vi "UnitTest.vi"() -> ()   [LabVIEW 2018]
doc: "This VI Tests the movement, and control of the Thorlab Axis Controller. You can use it to send any kind of configuration, or list of commands and verify things work properly.\n\nCreator: Slade Jeppesen\nCreated: 09/30/20"
uses:
  PPLs/Axis/Parent/Axis.lvlibp/Custom Controls/Command.ctl
  Thorlabs.lvclass
  PPLs/Axis/Parent/Axis.lvlibp/Custom Controls/Jog Direction.ctl
  PPLs/Axis/Parent/Axis.lvlibp/Axis.lvclass
  PPLs/Axis/Parent/Axis.lvlibp
  C:/AME Test Engineering/LabVIEW/PPLs/Axis/Parent/Axis.lvlibp/Axis.lvclass
panel:
  in  "PPLs Folder Path":path
  in  "INI File Path":path
  in  "Stop":bool
  in  "Jog Forwad":bool
  in  "Jog Back":bool
  in  "Step Back":bool
  in  "Step Forward":bool
  out "Error Out":errorcluster
  in  "Error In":errorcluster
  out "Current Position":dbl
  in  "Value":dbl
  out "Homed?":bool
  out "Moving?":bool
  out "Home Success?":bool
  in  "Command":T1
  in  "Home":bool
  in  "SendCMD":bool
  in  "Device":string
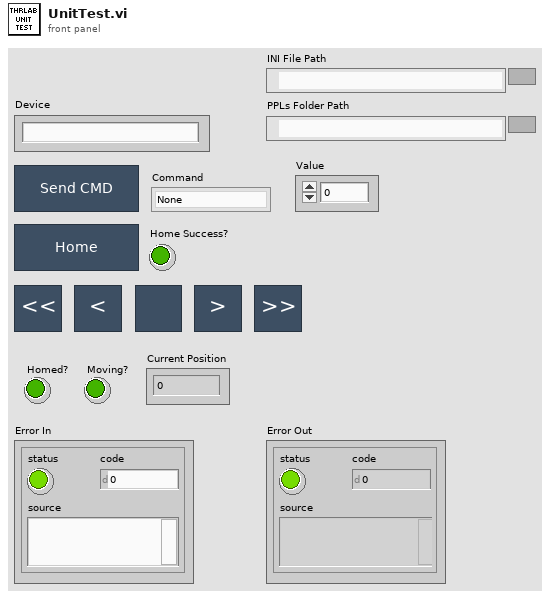
[diagram p1: front panel]
types:
  T1 = typedef "Axis.lvlibp/Command.ctl" = enum16{"None", "Home", "Renumber", "Move Absolute", "Move Relative", "Stop", "Set Run Speed", "Set Acceleration", "Set Run Current", "Set Home Offset", "Set Home Speed", "Query Current Position", "Load Defaults", "Query Status", "Lock Controls", "Unlock Controls", "Set Jog Step Size", "Set Jog Acceleration", "Set Jog Speed", "Query Homed Status", "Query Moving Status", "Reset", "Set Max Position", "Set Min Position"}
  T2 = typedef "Axis.lvlibp/Jog Direction.ctl" = enum16{"Forward", "Backward"}
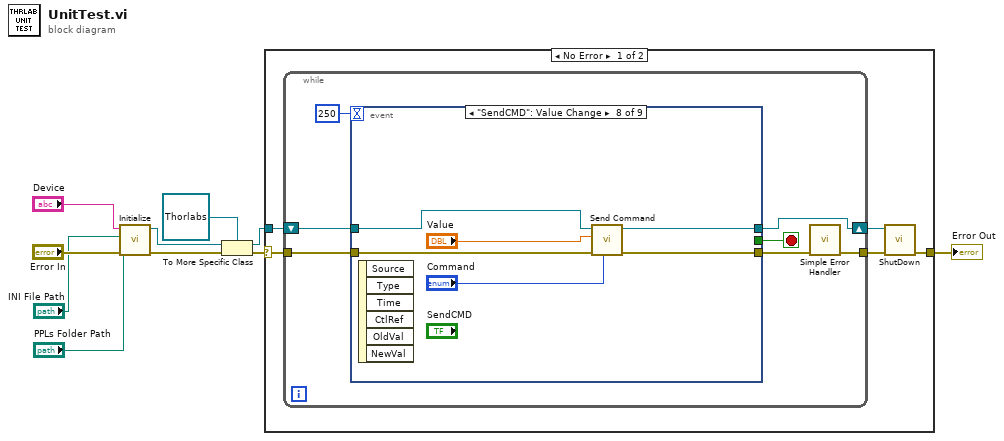
[diagram p0: block diagram]
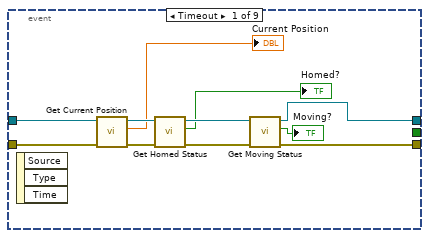
[diagram p2: hidden frame]
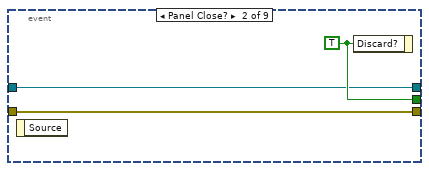
[diagram p3: hidden frame]
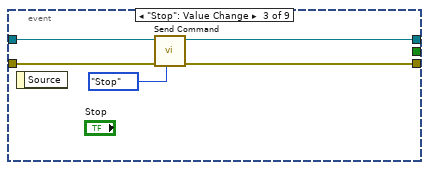
[diagram p4: hidden frame]
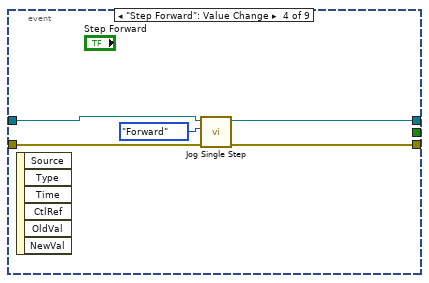
[diagram p5: hidden frame]
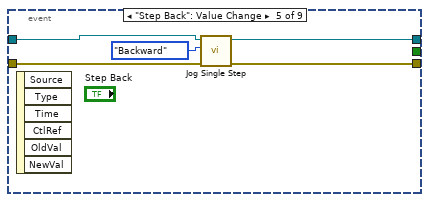
[diagram p6: hidden frame]
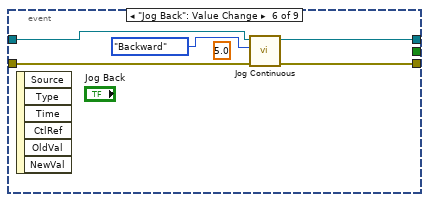
[diagram p7: hidden frame]
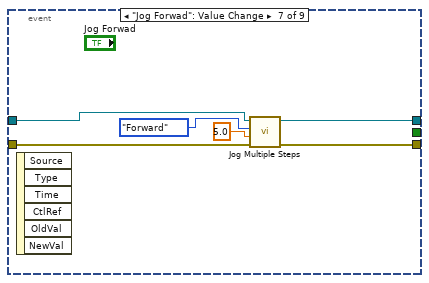
[diagram p8: hidden frame]
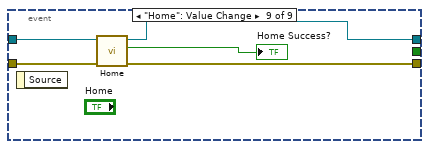
[diagram p9: hidden frame]
diagram:
  n1 = call "Initialize.vi"("error in"="Error In", "PPLs Folder Path"="PPLs Folder Path", "INI File Path"="INI File Path", "Device"="Device") -> ("error out"=w8:errorcluster, "Axis out"=w10:refnum<class "Axis.lvclass">)  [unwired: 6 in]
  n2 = To More Specific Class(target class=refnum<class "Thorlabs.lvclass"> refnum ("Thorlabs.lvlib:Thorlabs.lvclass"), reference=w10, error in=w8) -> (specific class reference=w7:refnum<class "Thorlabs.lvclass">, error out=w6:errorcluster)
  n3 = case shown="No Error" w6 {
    selector: w6 -> [w11 w74]
    tunnel: w7 -> [w15 _]
    tunnel: [w13 w74] -> w4
    frame No Error {
      n4 = while {
        shift-right: [w19] -> w14
        shift-left: w15 -> [w20]
        tunnel: w11 -> [w21]
        tunnel: [w17] -> w12
        stop <- w22 stop-if-true
        n5 = event shown="[7] \"SendCMD\": Value Change" {
          selector: _ -> [_ _ _ _ _ _ _ _ _]
          dyn-events: _ -> [_ _ _ _ _ _ _ _ _]
          timeout: 250 -> [_ _ _ _ _ _ _ _ _]
          tunnel: [_ w36 _ _ _ _ _ _ _] -> w22
          tunnel: w21 -> [w26 w34 w40 w46 w51 w55 w59 w65 w73]
          tunnel: w20 -> [w23 w35 w37 w45 w50 w52 w60 w68 w72]
          tunnel: [w24 w35 w38 w43 w49 w53 w57 w67 w71] -> w19
          tunnel: [w25 w34 w39 w42 w48 w54 w58 w66 w70] -> w18
          event Timeout {
            n6 = event-data() -> ()  [unwired: 1 in, 3 out]
            n7 = call "Get Current Position.vi"("error in"=w26, "Axis in"=w23) -> ("error out"=w31:errorcluster, "Current Position"=→"Current Position":dbl, "Axis out"=w33:refnum<class "Thorlabs.lvclass">)  [unwired: 7 in]
            n8 = call "Get Homed Status.vi"("error in (no error)"=w31, "Axis in"=w33) -> ("error out"=w30:errorcluster, "Homed?"=→"Homed?":bool, "Axis out"=w32:refnum<class "Thorlabs.lvclass">)  [unwired: 7 in]
            n9 = call "Get Moving Status.vi"("error in (no error)"=w30, "Axis in"=w32) -> ("error out"=w25:errorcluster, "Moving?"=→"Moving?":bool, "Axis out"=w24:refnum<class "Thorlabs.lvclass">)  [unwired: 7 in]
          }
          event Panel Close? {
            w36 = TRUE
            n10 = event-data() -> ()  [unwired: 1 in, 1 out]
            n11 = event-data("Discard?"=w36) -> ()  [unwired: 1 in, 1 out]
          }
          event "Stop": Value Change {
            n12 = event-data() -> ()  [unwired: 1 in, 1 out]
            n13 = call-dynamic "Send Command.vi"("Command"=Command."Stop", "error in"=w40, "Thorlabs In"=w37) -> ("error out"=w39:errorcluster, "Thorlabs Out"=w38:refnum<class "Thorlabs.lvclass">)  [unwired: 7 in]
          }
          event "Step Forward": Value Change {
            n14 = event-data() -> ()  [unwired: 1 in, 6 out]
            n15 = call-dynamic "Jog Single Step.vi"("error in (no error)"=w46, "Jog Direction"=Jog_Direction."Forward", "Thorlabs in"=w45) -> ("error out"=w42:errorcluster, "Thorlabs out"=w43:refnum<class "Thorlabs.lvclass">)  [unwired: 7 in]
          }
          event "Step Back": Value Change {
            n16 = event-data() -> ()  [unwired: 1 in, 6 out]
            n17 = call-dynamic "Jog Single Step.vi"("error in (no error)"=w51, "Jog Direction"=Jog_Direction."Backward", "Thorlabs in"=w50) -> ("error out"=w48:errorcluster, "Thorlabs out"=w49:refnum<class "Thorlabs.lvclass">)  [unwired: 7 in]
          }
          event "Jog Back": Value Change {
            (unwired) 5.0 ("StepAmount")
            n18 = event-data() -> ()  [unwired: 1 in, 6 out]
            n19 = call-dynamic "Jog Continuous.vi"("error in (no error)"=w55, "Jog Direction"=Jog_Direction."Backward", "Thorlabs in"=w52) -> ("error out"=w54:errorcluster, "Thorlabs out"=w53:refnum<class "Thorlabs.lvclass">)  [unwired: 7 in]
          }
          event "Jog Forwad": Value Change {
            n20 = event-data() -> ()  [unwired: 1 in, 6 out]
            n21 = call-dynamic "Jog Multiple Steps.vi"("error in (no error)"=w59, "StepAmount"=5.0, "Jog Direction"=Jog_Direction."Forward", "Thorlabs in"=w60) -> ("error out"=w58:errorcluster, "Thorlabs out"=w57:refnum<class "Thorlabs.lvclass">)  [unwired: 6 in]
          }
          event "SendCMD": Value Change {
            n22 = event-data() -> ()  [unwired: 1 in, 6 out]
            n23 = call-dynamic "Send Command.vi"("Command"="Command", "error in"=w65, "Value"="Value", "Thorlabs In"=w68) -> ("error out"=w66:errorcluster, "Thorlabs Out"=w67:refnum<class "Thorlabs.lvclass">)  [unwired: 6 in]
          }
          event "Home": Value Change {
            n24 = event-data() -> ()  [unwired: 1 in, 1 out]
            n25 = call "Home.vi"("error in"=w73, "Axis in"=w72) -> ("error out"=w70:errorcluster, "Success?"=→"Home Success?":bool, "Axis out"=w71:refnum<class "Thorlabs.lvclass">)  [unwired: 7 in]
          }
        }
        n26 = call <vilib>:"Simple Error Handler.vi"("error in (no error)"=w18) -> ("error out"=w17:errorcluster)  [unwired: 4 in, 4 out]
      }
      n27 = call "ShutDown.vi"("error in"=w12, "Axis in"=w14) -> ("error out"=w13:errorcluster)  [unwired: 8 in, 1 out]
    }
    frame Error {
    }
  }
  "Error Out" <- w4
